vi "CRYAPI MARK LIB.vi"(0 "sAction":string="asada", 2 "Docking_Update":bool=TRUE, 3 "MousePos":T2) -> (9 "Rect_Out":T1, 10 "bResult":bool=TRUE)   [LabVIEW 2013]
uses:
  <vilib>/Utility/miscctls.llb/LVRectTypeDef.ctl
  CRYMain Sub Window Global.vi
panel:
  in  "Rect_SUB":T1[](array[typedef])
  in  "Rect_LRAB":T1[](array[typedef])
  in  "Rect_Main":T1
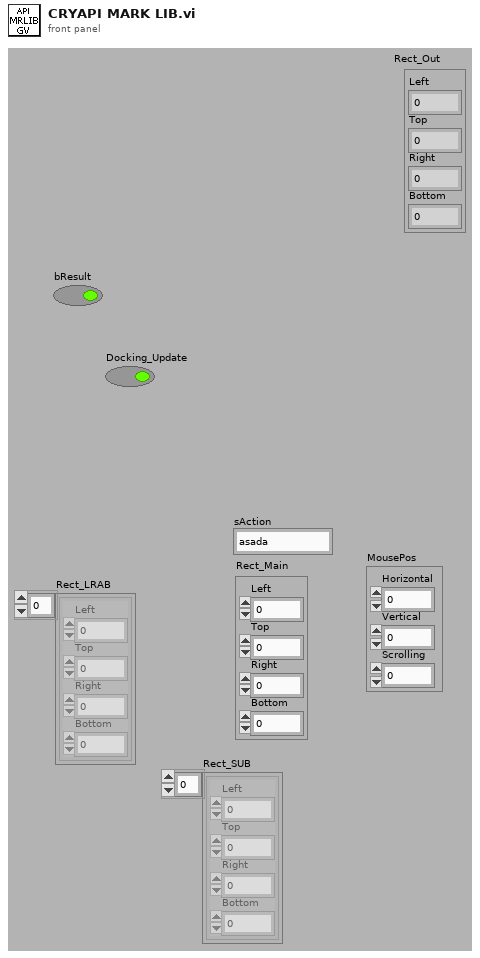
[diagram p1: front panel]
types:
  T1 = typedef "LVRectTypeDef.ctl" = cluster{"Left":i16, "Top":i16, "Right":i16, "Bottom":i16}
  T2 = cluster{"Horizontal":i32, "Vertical":i32, "Scrolling":i32}
  T3 = enum32{"Invalid", "Standard", "Closed", "Hidden", "Minimized", "Maximized"}
  T4 = enum32{"Invalid", "Default", "Floating", "Floating/Auto-Hide", "Modal"}
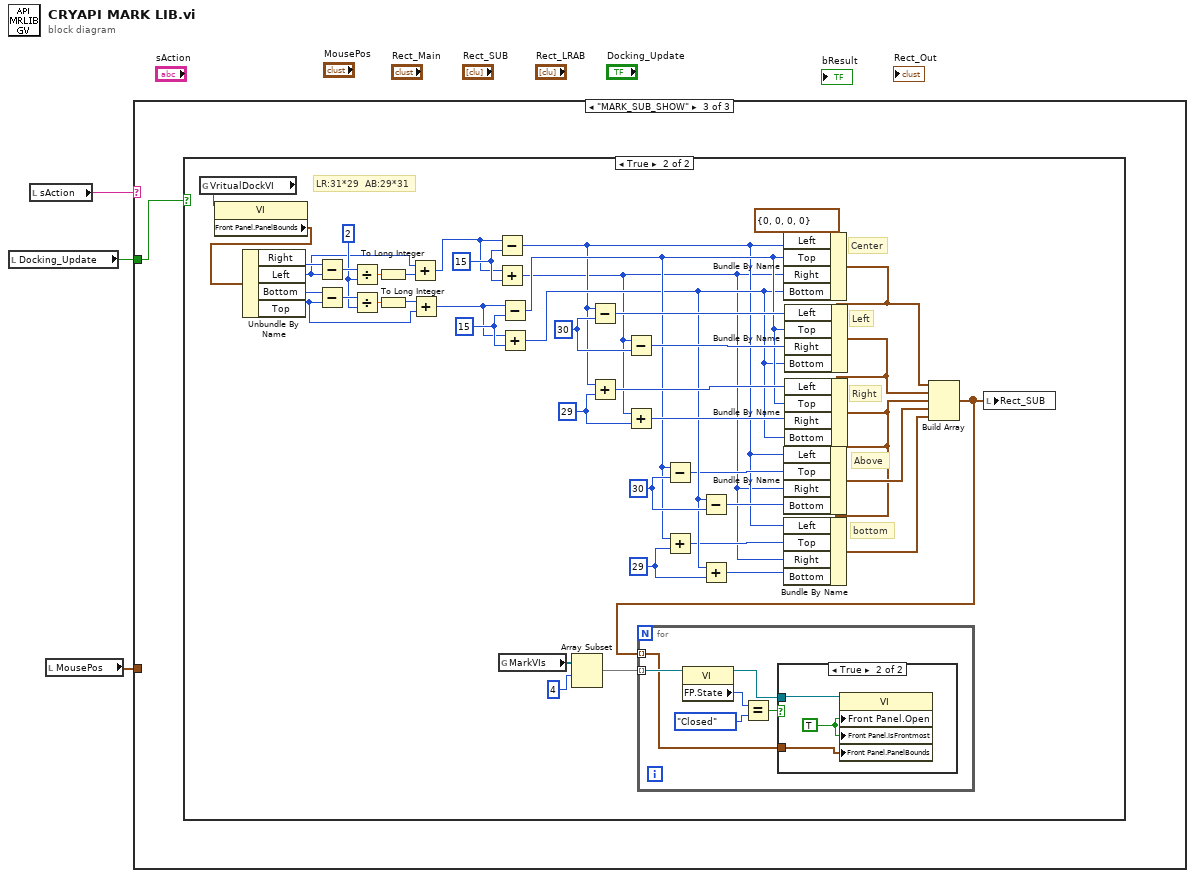
[diagram p0: block diagram]
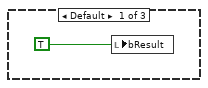
[diagram p2: hidden frame]
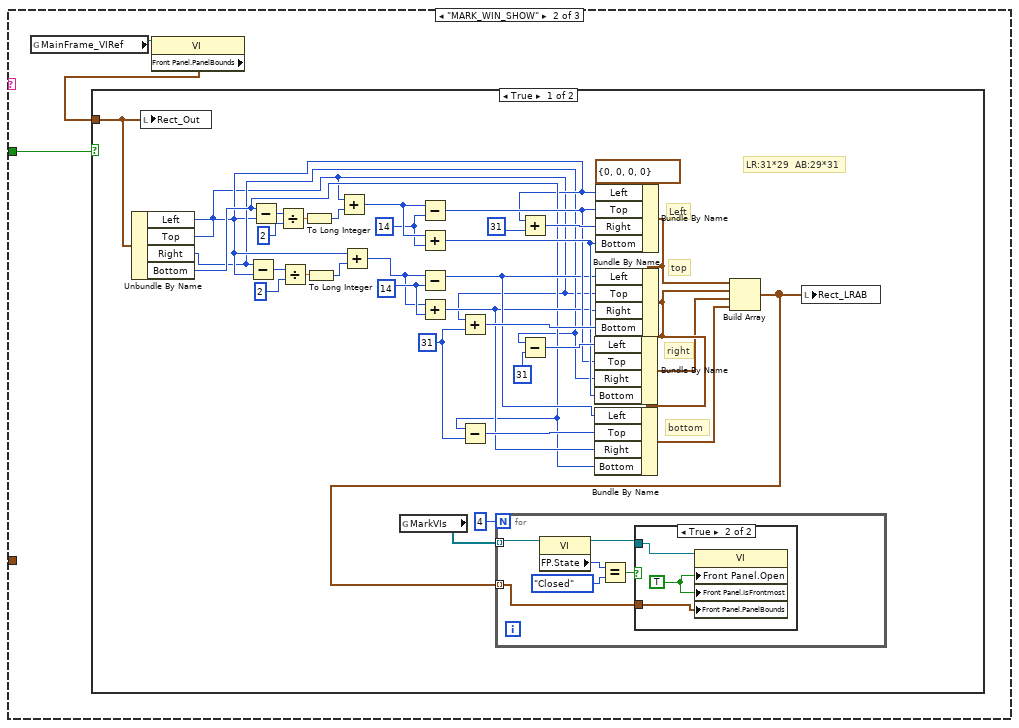
[diagram p3: hidden frame]
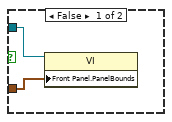
[diagram p4: hidden frame]
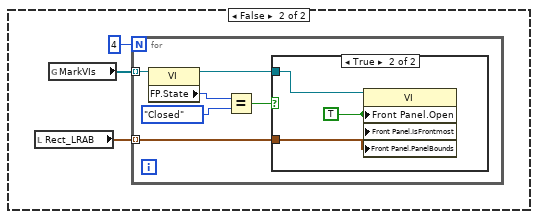
[diagram p5: hidden frame]
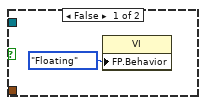
[diagram p6: hidden frame]
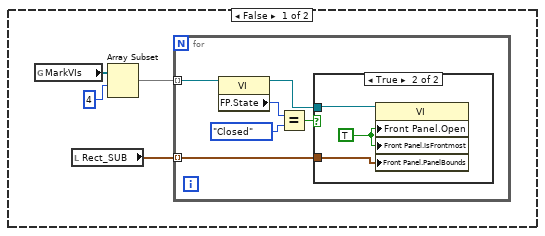
[diagram p7: hidden frame]
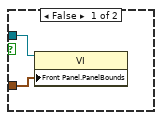
[diagram p8: hidden frame]
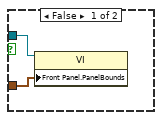
[diagram p9: hidden frame]
diagram:
  n1 = local read "Docking_Update"() -> (w1:bool)
  n2 = local read "sAction"() -> (w3:string)
  n3 = local read "MousePos"() -> (w2:T2)
  n4 = case shown="\"MARK_SUB_SHOW\"" w3 {
    tunnel: w2 -> [_ _ _]
    tunnel: w1 -> [_ w5 w68]
    frame Default {
      n5 = local write "bResult"(TRUE ("bResult")) -> ()
    }
    frame "MARK_WIN_SHOW" {
      n6 = global read "CRYMain Sub Window Global.vi" "MainFrame_VIRef"() -> (w7:refnum<vi>)
      n7 = property class="VI"(reference=w7) -> ("Front Panel.PanelBounds"=w6:T1)  [unwired: 1 in, 2 out]
      n8 = case shown="True" w5 {
        tunnel: w6 -> [w8 _]
        frame True {
          w25 = 14
          w32 = 31
          w28 = 14
          # "LR:31*29  AB:29*31"
          # "bottom"
          # "right"
          # "top"
          # "Left"
          n9 = Unbundle By Name(w8) -> ("Left"=w17:i16, "Top"=w13:i16, "Right"=w16:i16, "Bottom"=w20:i16)
          n10 = local write "Rect_Out"(w8) -> ()
          n11 = Subtract(x=w16, y=w17) -> (x-y=w35:i16)
          n12 = Subtract(x=w20, y=w13) -> (x-y=w12:i16)
          n13 = Divide(x=w12, y=2) -> (x/y=w10:dbl)
          n14 = Divide(x=w35, y=2) -> (x/y=w15:dbl)
          n15 = To Long Integer(number=w10) -> (32bit integer=w9:i32)
          n16 = To Long Integer(number=w15) -> (32bit integer=w14:i32)
          n17 = Add(x=w13, y=w9) -> (x+y=w29:i32)
          n18 = Add(x=w17, y=w14) -> (x+y=w24:i32)
          n19 = global read "CRYMain Sub Window Global.vi" "MarkVIs"() -> (w39:refnum<vi>[])
          n20 = Subtract(x=w29, y=w28) -> (x-y=w26:i32)
          n21 = Add(x=w29, y=w28) -> (x+y=w27:i32)
          n22 = Subtract(x=w24, y=w25) -> (x-y=w23:i32)
          n23 = Add(x=w24, y=w25) -> (x+y=w22:i32)
          n24 = Add(x=w13, y=w32) -> (x+y=w33:i32)
          n25 = Subtract(x=w20, y=w32) -> (x-y=w31:i32)
          n26 = Add(x=w17, y=31) -> (x+y=w30:i32)
          n27 = Subtract(x=w16, y=31) -> (x-y=w34:i32)
          n28 = Bundle By Name(cluster=T1 {"Left"=0, "Top"=0, "Right"=0, "Bottom"=0} ("Front Panel Window:Panel Bounds"), "Left"=w17, "Top"=w26, "Right"=w30, "Bottom"=w27) -> (w43:T1)
          n29 = Bundle By Name(cluster=w43, "Left"=w23, "Top"=w13, "Right"=w22, "Bottom"=w33) -> (w42:T1)
          n30 = Bundle By Name(cluster=w42, "Left"=w34, "Top"=w26, "Right"=w16, "Bottom"=w27) -> (w41:T1)
          n31 = Bundle By Name(cluster=w42, "Left"=w23, "Top"=w31, "Right"=w22, "Bottom"=w20) -> (w40:T1)
          n32 = Build Array(w43, w42, w41, w40) -> (w11:T1[])
          n33 = for {
            N: 4 -> [_]
            tunnel: w11 -> [w44] mode=indexing
            tunnel: w39 -> [w49] mode=indexing
            n34 = property class="VI"(reference=w49) -> (reference out=w48:refnum<vi>, "FP.State"=w47:T3)  [unwired: 1 in, 1 out]
            n35 = Equal?(x=w47, y=T3."Closed" ("Front Panel Window:State")) -> (x = y?=w45:bool)
            n36 = case shown="True" w45 {
              tunnel: w48 -> [w51 w52]
              tunnel: w44 -> [w50 w54]
              frame False {
                n37 = property class="VI"(reference=w51, "Front Panel.PanelBounds"=w50) -> ()  [unwired: 1 in, 2 out]
              }
              frame True {
                w53 = TRUE ("Front Panel Window:Open")
                n38 = property class="VI"(reference=w52, "Front Panel.Open"=w53, "Front Panel.IsFrontmost"=w53, "Front Panel.PanelBounds"=w54) -> ()  [unwired: 1 in, 2 out]
              }
            }
          }
          n39 = local write "Rect_LRAB"(w11) -> ()
        }
        frame False {
          n40 = local read "Rect_LRAB"() -> (w55:T1[])
          n41 = global read "CRYMain Sub Window Global.vi" "MarkVIs"() -> (w57:refnum<vi>[])
          n42 = for {
            N: 4 -> [_]
            tunnel: w57 -> [w60] mode=indexing
            tunnel: w55 -> [w58] mode=indexing
            n43 = property class="VI"(reference=w60) -> (reference out=w59:refnum<vi>, "FP.State"=w63:T3)  [unwired: 1 in, 1 out]
            n44 = Equal?(x=w63, y=T3."Closed" ("Front Panel Window:State")) -> (x = y?=w61:bool)
            n45 = case shown="True" w61 {
              tunnel: w59 -> [_ w67]
              tunnel: w58 -> [_ w65]
              frame False {
                n46 = property class="VI"("FP.Behavior"=T4."Floating" ("Front Panel Window:Behavior")) -> ()  [unwired: 2 in, 2 out]
              }
              frame True {
                w66 = TRUE ("Front Panel Window:Open")
                n47 = property class="VI"(reference=w67, "Front Panel.Open"=w66, "Front Panel.IsFrontmost"=w66, "Front Panel.PanelBounds"=w65) -> ()  [unwired: 1 in, 2 out]
              }
            }
          }
        }
      }
    }
    frame "MARK_SUB_SHOW" {
      n48 = case shown="True" w68 {
        frame False {
          n49 = global read "CRYMain Sub Window Global.vi" "MarkVIs"() -> (w71:refnum<vi>[])
          n50 = local read "Rect_SUB"() -> (w69:T1[])
          n51 = Array Subset(array=w71, index=4) -> (w72:refnum<vi>[])  [unwired: 1 in]
          n52 = for {
            tunnel: w72 -> [w74] mode=indexing
            tunnel: w69 -> [w73] mode=indexing
            n53 = property class="VI"(reference=w74) -> (reference out=w75:refnum<vi>, "FP.State"=w76:T3)  [unwired: 1 in, 1 out]
            n54 = Equal?(x=w76, y=T3."Closed" ("Front Panel Window:State")) -> (x = y?=w78:bool)
            n55 = case shown="True" w78 {
              tunnel: w75 -> [w80 w82]
              tunnel: w73 -> [w79 w81]
              frame False {
                n56 = property class="VI"(reference=w80, "Front Panel.PanelBounds"=w79) -> ()  [unwired: 1 in, 2 out]
              }
              frame True {
                w83 = TRUE ("Front Panel Window:Open")
                n57 = property class="VI"(reference=w82, "Front Panel.Open"=w83, "Front Panel.IsFrontmost"=w83, "Front Panel.PanelBounds"=w81) -> ()  [unwired: 1 in, 2 out]
              }
            }
          }
        }
        frame True {
          w84 = 29
          w85 = 29
          w97 = 30
          w109 = 15
          w100 = 30
          w123 = 15
          w112 = 2
          # "Center"
          # "LR:31*29  AB:29*31"
          # "bottom"
          # "Above"
          # "Right"
          # "Left"
          n58 = global read "CRYMain Sub Window Global.vi" "VritualDockVI"() -> (w125:refnum<vi>)
          n59 = property class="VI"(reference=w125) -> ("Front Panel.PanelBounds"=w118:T1)  [unwired: 1 in, 2 out]
          n60 = Unbundle By Name(w118) -> ("Right"=w117:i16, "Left"=w107:i16, "Bottom"=w115:i16, "Top"=w106:i16)
          n61 = Subtract(x=w117, y=w107) -> (x-y=w116:i16)
          n62 = Subtract(x=w115, y=w106) -> (x-y=w113:i16)
          n63 = Divide(x=w116, y=w112) -> (x/y=w124:dbl)
          n64 = Divide(x=w113, y=w112) -> (x/y=w114:dbl)
          n65 = To Long Integer(number=w124) -> (32bit integer=w108:i32)
          n66 = To Long Integer(number=w114) -> (32bit integer=w105:i32)
          n67 = Add(x=w107, y=w108) -> (x+y=w104:i32)
          n68 = Add(x=w105, y=w106) -> (x+y=w103:i32)
          n69 = Subtract(x=w104, y=w109) -> (x-y=w90:i32)
          n70 = Add(x=w104, y=w109) -> (x+y=w89:i32)
          n71 = global read "CRYMain Sub Window Global.vi" "MarkVIs"() -> (w88:refnum<vi>[])
          n72 = Subtract(x=w103, y=w123) -> (x-y=w96:i32)
          n73 = Add(x=w103, y=w123) -> (x+y=w95:i32)
          n74 = Array Subset(array=w88, index=4) -> (w87:refnum<vi>[])  [unwired: 1 in]
          n75 = Subtract(x=w90, y=w100) -> (x-y=w102:i32)
          n76 = Add(x=w90, y=w85) -> (x+y=w99:i32)
          n77 = Subtract(x=w89, y=w100) -> (x-y=w101:i32)
          n78 = Add(x=w89, y=w85) -> (x+y=w98:i32)
          n79 = Subtract(x=w96, y=w97) -> (x-y=w94:i32)
          n80 = Add(x=w96, y=w84) -> (x+y=w92:i32)
          n81 = Subtract(x=w95, y=w97) -> (x-y=w93:i32)
          n82 = Add(x=w95, y=w84) -> (x+y=w91:i32)
          n83 = Bundle By Name(cluster=T1 {"Left"=0, "Top"=0, "Right"=0, "Bottom"=0} ("Front Panel Window:Panel Bounds"), "Left"=w90, "Top"=w96, "Right"=w89, "Bottom"=w95) -> (w110:T1)
          n84 = Bundle By Name(cluster=w110, "Left"=w102, "Top"=w96, "Right"=w101, "Bottom"=w95) -> (w119:T1)
          n85 = Bundle By Name(cluster=w119, "Left"=w99, "Top"=w96, "Right"=w98, "Bottom"=w95) -> (w120:T1)
          n86 = Bundle By Name(cluster=w120, "Left"=w90, "Top"=w94, "Right"=w89, "Bottom"=w93) -> (w121:T1)
          n87 = Bundle By Name(cluster=w120, "Left"=w90, "Top"=w92, "Right"=w89, "Bottom"=w91) -> (w122:T1)
          n88 = Build Array(w110, w119, w120, w121, w122) -> (w86:T1[])
          n89 = for {
            tunnel: w87 -> [w128] mode=indexing
            tunnel: w86 -> [w127] mode=indexing
            n90 = property class="VI"(reference=w128) -> (reference out=w129:refnum<vi>, "FP.State"=w130:T3)  [unwired: 1 in, 1 out]
            n91 = Equal?(x=w130, y=T3."Closed" ("Front Panel Window:State")) -> (x = y?=w132:bool)
            n92 = case shown="True" w132 {
              tunnel: w129 -> [w134 w136]
              tunnel: w127 -> [w133 w135]
              frame False {
                n93 = property class="VI"(reference=w134, "Front Panel.PanelBounds"=w133) -> ()  [unwired: 1 in, 2 out]
              }
              frame True {
                w137 = TRUE ("Front Panel Window:Open")
                n94 = property class="VI"(reference=w136, "Front Panel.Open"=w137, "Front Panel.IsFrontmost"=w137, "Front Panel.PanelBounds"=w135) -> ()  [unwired: 1 in, 2 out]
              }
            }
          }
          n95 = local write "Rect_SUB"(w86) -> ()
        }
      }
    }
  }
